vi "IR_Correction.vi"(1 "X Rate":bool=TRUE, 2 "X_Rotate Rate":bool=TRUE, 3 "Y Rate":bool=TRUE, 4 "Y_Rotate Rate":bool=TRUE, 5 "Mode":enum16{"LF", "LB", "RF", "RB"}(ring), 11 "error in":errorcluster, 12 "width":bool) -> (15 "error out":errorcluster)   [LabVIEW 2019]
uses:
  <vilib>/Platform/TimedLoop/XDataNode/timing_clust.ctl
  <vilib>/Platform/TimedLoop/XDataNode/nitl_modes.ctl
  <vilib>/Platform/TimedLoop/XDataNode/wakeup.ctl
  WSCbot_V3_Toolkit.lvlibp/WSCBOTV3_Toolkit/Sensor/LowLevel/IR_Chanel.ctl
  WSCbot_V3_Toolkit.lvlibp/WSCBOTV3_Toolkit/System/LowLevel/EMS.vi
  <vilib>/platform/TimedLoop/XDataNode/XDataNode.xnode
  <vilib>/Platform/TimedLoop/XDataNode/XDNodeRunTimeDep.lvlib
  WSCbot_V3_Toolkit.lvlibp
panel:
  out "X_Rotate IR":bool
  out "X_Rotate IR":dbl
  in  "Power Rate":dbl
  out "4xMotor":dbl[](graph)
  out "ENC":dbl[](graph)
  out "Waveform Chart 2":T1(graph)
  out "IR":T2
  out "Y_Rotate IR":dbl
  out "X Position IR":dbl
  out "Y Position IR":dbl
  out "Y_Rotate IR":bool
  out "X Position IR":bool
  out "Y Position IR":bool
  in  "Stop":bool
  out "result":bool
  out "Numeric":i32
  out "coerced(x)":dbl
  out "Boolean":bool
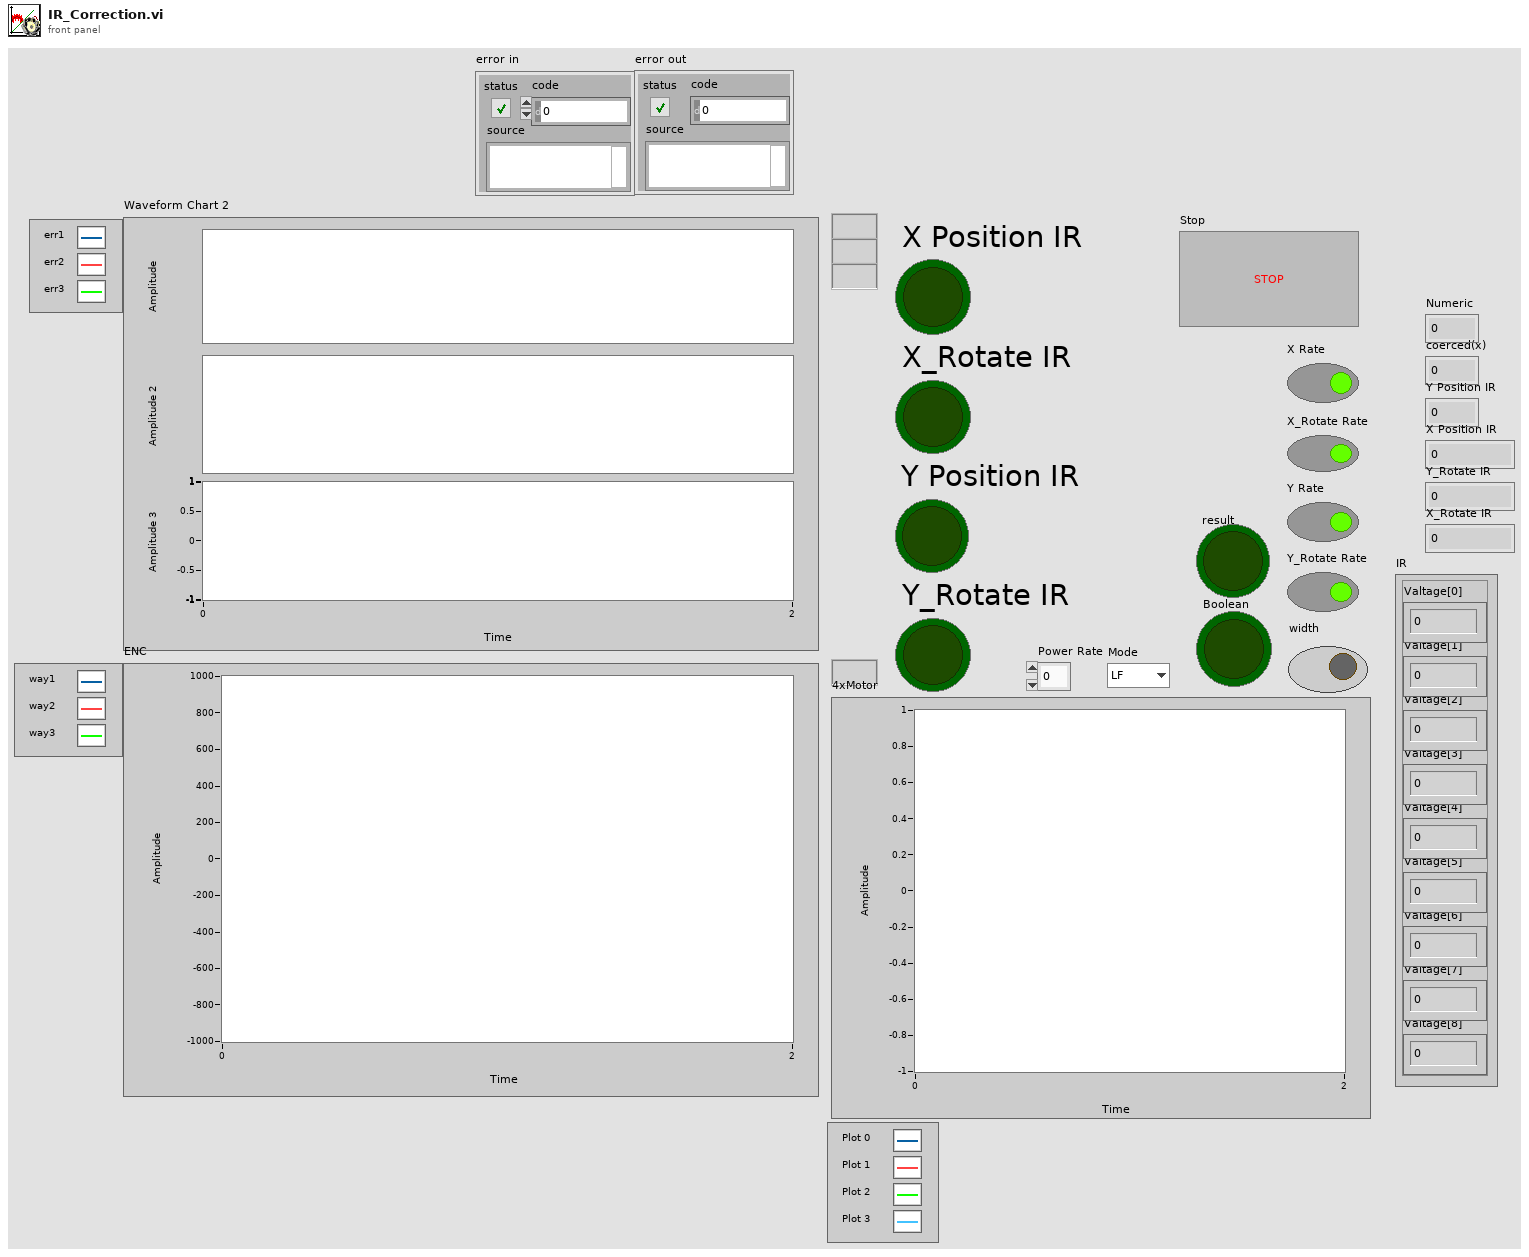
[diagram p1: front panel]
types:
  T1 = cluster{"Valtage[0]":dbl, "Valtage[1]":dbl, "Valtage[2]":dbl}
  T2 = cluster{"Valtage[0]":dbl, "Valtage[1]":dbl, "Valtage[2]":dbl, "Valtage[3]":dbl, "Valtage[4]":dbl, "Valtage[5]":dbl, "Valtage[6]":dbl, "Valtage[7]":dbl, "Valtage[8]":dbl}
  T3 = typedef "WSCbot_V3_Toolkit.lvlibp/IR_Chanel.ctl" = enum16{"IR_LF", "IR_LB", "IR_BL", "IR_BR", "IR_RB", "IR_RF", "IR_FR", "IR_FL"}
  T4 = typedef "XDNodeRunTimeDep.lvlib/timing_clust.ctl" = cluster{"Expected End [f-1]":u64, "Actual End [f-1]":u64, "Finished Late? [f-1]":bool, "Expected End [i-1]":u64, "Actual End [i-1]":u64, "Finished Late? [i-1]":bool, "Expected Start [i]":u64, "Actual Start [i]":u64, "Expected Start [f]":u64, "Actual Start [f]":u64, "Source Name":string, "Structure Name":string, "Period":i64, "Deadline":i64, "Offset":i64, "Start":i64, "Priority":i32, "Timeout":i32, "Mode":T5, "Wakeup Reason":T6, "Error":errorcluster, "Source Type":string, "Secondary Source Type":string, "Global End Time":u64, "Global Start Time":u64, "Frame Duration":u64, "Iteration Duration":u64, "Assigned CPU":i32, "I/O Scan Engine Mode":u32}
  T5 = typedef "XDNodeRunTimeDep.lvlib/nitl_modes.ctl" = enum32{"No Change", "Process missed periods, maintain original phase", "Discard missed periods, maintain original phase", "Process missed periods, ignore original phase", "Discard missed periods, ignore original phase"}
  T6 = typedef "XDNodeRunTimeDep.lvlib/wakeup.ctl" = enum32{"Normal", "Aborted", "Asynchronous wakeup", "Timing source error", "Timed loop error", "Timeout"}
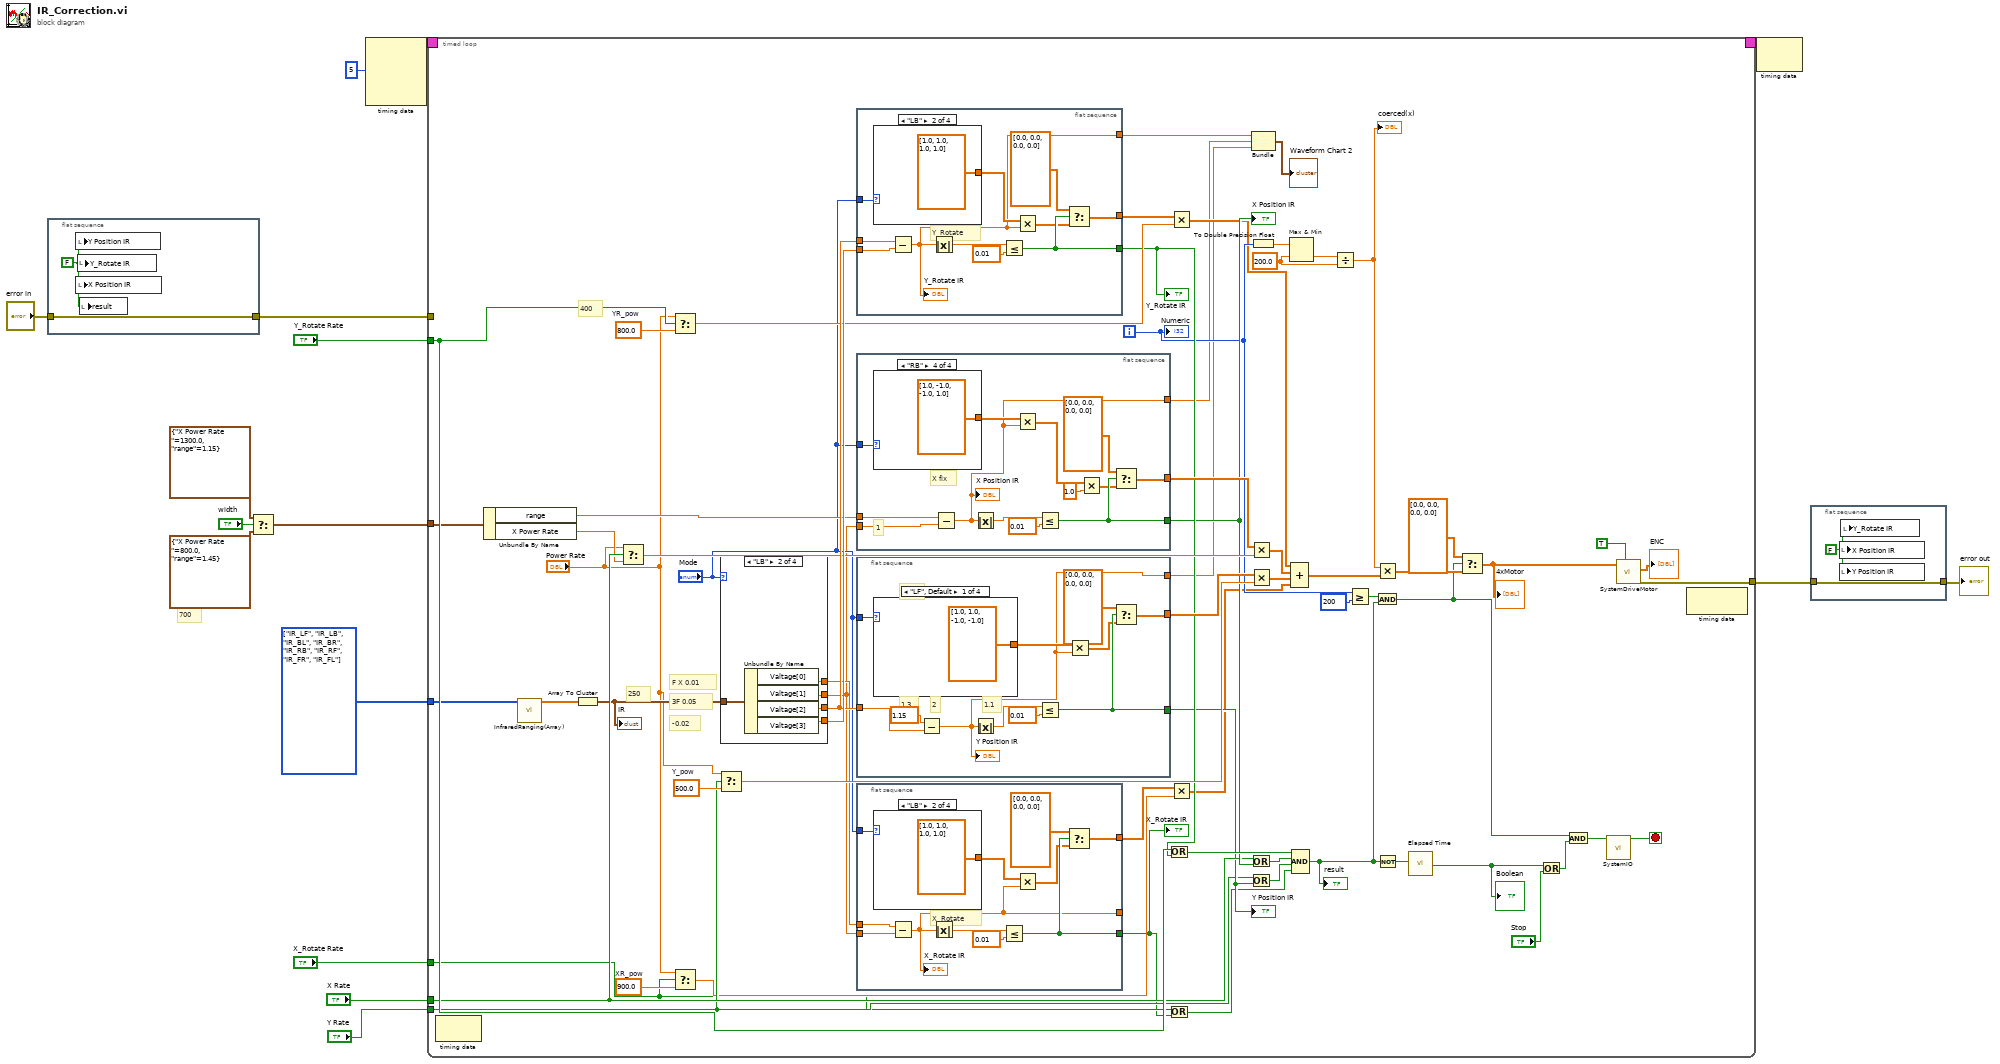
[diagram p0: block diagram]
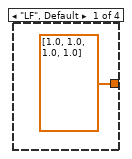
[diagram p2: hidden frame]
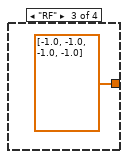
[diagram p3: hidden frame]
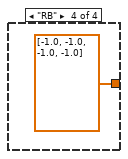
[diagram p4: hidden frame]
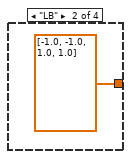
[diagram p5: hidden frame]
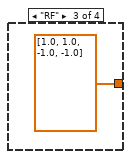
[diagram p6: hidden frame]
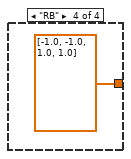
[diagram p7: hidden frame]
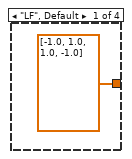
[diagram p8: hidden frame]
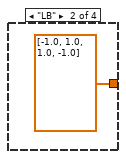
[diagram p9: hidden frame]
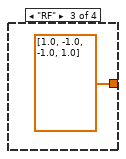
[diagram p10: hidden frame]
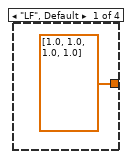
[diagram p11: hidden frame]
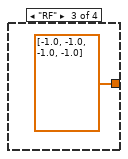
[diagram p12: hidden frame]
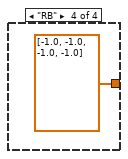
[diagram p13: hidden frame]
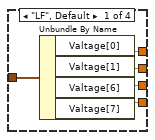
[diagram p14: hidden frame]
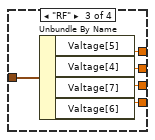
[diagram p15: hidden frame]
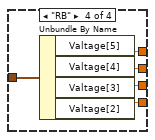
[diagram p16: hidden frame]
diagram:
  w4 = T3[] [enum."IR_LF", enum."IR_LB", enum."IR_BL", enum."IR_BR", enum."IR_RB", enum."IR_RF", enum."IR_FR", enum."IR_FL"] items=["IR_LF", "IR_LB", "IR_BL", "IR_BR", "IR_RB", "IR_RF", "IR_FR", "IR_FL"] ("IR_Chanel")
  # "700"
  n1 = flat-sequence {
    tunnel: "error in" -> [w18]
    tunnel: [w18] -> w3
    frame #0 {
      w17 = FALSE
      n2 = local write "Y Position IR"(w17) -> ()
      n3 = local write "X Position IR"(w17) -> ()
      n4 = local write "Y_Rotate IR"(w17) -> ()
      n5 = local write "result"(w17) -> ()
    }
  }
  n6 = Select(t=cluster{"X Power Rate ":dbl, "range":dbl} {"X Power Rate "=1300.0, "range"=1.15}, s="width", f=cluster{"X Power Rate ":dbl, "range":dbl} {"X Power Rate "=800.0, "range"=1.45}) -> (s? t:f=w8:cluster{"X Power Rate ":dbl, "range":dbl})
  n7 = node-c288(i64 5 ("Period")) -> (w16:T4)  [unwired: 3 in]
  n8 = timed-loop {
    timing: w16 -> [_]
    timing-out: [_] -> w15
    tunnel: w3 -> [_]
    tunnel: [w51] -> w1
    tunnel: "Y_Rotate Rate" -> [w65]
    tunnel: "X Rate" -> [w61]
    tunnel: "Y Rate" -> [w58]
    tunnel: w8 -> [w56]
    tunnel: w4 -> [w45]
    tunnel: "X_Rotate Rate" -> [w21]
    i -> [w40]
    stop <- w50 stop-if-true
    w28 = 900.0  # XR_pow
    w42 = 200.0 ("y")
    w67 = 500.0  # Y_pow
    w70 = 800.0  # YR_pow
    # "250"
    # "400"
    # "3F 0.05"
    # "F X 0.01"
    # "-0.02"
    n9 = node-c288() -> ()  [unwired: 1 in, 1 out]
    n10 = Unbundle By Name(w56) -> ("range"=w55:dbl, "X Power Rate"=w54:dbl)
    n11 = call "InfraredRanging(Array).vi"("IR_Chanel"=w45) -> ("Valtage"=w47:dbl[])  [unwired: 9 in, 1 out]
    n12 = Array To Cluster(array=w47) -> (cluster=w46:T2)
    "IR" <- w46
    n13 = Select(t="Power Rate", s=w61, f=w54) -> (s? t:f=w68:dbl)
    n14 = Select(t="Power Rate", s=w65, f=w70) -> (s? t:f=w69:dbl)
    n15 = Select(t="Power Rate", s=w21, f=w28) -> (s? t:f=w27:dbl)
    n16 = Select(t="Power Rate", s=w58, f=w67) -> (s? t:f=w66:dbl)
    n17 = case shown="\"LB\"" "Mode" {
      tunnel: [w150 w155 w159 w164] -> w82
      tunnel: [w149 w154 w160 w165] -> w83
      tunnel: [w152 w156 w161 w166] -> w23
      tunnel: w46 -> [w151 w157 w162 w167]
      tunnel: [w148 w153 w158 w163] -> w24
      frame "LF", Default {
        n18 = Unbundle By Name(w151) -> ("Valtage[0]"=w148:dbl, "Valtage[1]"=w152:dbl, "Valtage[6]"=w150:dbl, "Valtage[7]"=w149:dbl)
      }
      frame "LB" {
        n19 = Unbundle By Name(w157) -> ("Valtage[0]"=w153:dbl, "Valtage[1]"=w156:dbl, "Valtage[2]"=w155:dbl, "Valtage[3]"=w154:dbl)
      }
      frame "RF" {
        n20 = Unbundle By Name(w162) -> ("Valtage[5]"=w158:dbl, "Valtage[4]"=w161:dbl, "Valtage[7]"=w159:dbl, "Valtage[6]"=w160:dbl)
      }
      frame "RB" {
        n21 = Unbundle By Name(w167) -> ("Valtage[5]"=w163:dbl, "Valtage[4]"=w166:dbl, "Valtage[3]"=w164:dbl, "Valtage[2]"=w165:dbl)
      }
    }
    n22 = flat-sequence {
      tunnel: w82 -> [w141]
      tunnel: w83 -> [w140]
      tunnel: "Mode" -> [w139]
      tunnel: [w137] -> w64
      tunnel: [w134] -> w81
      tunnel: [w131] -> w36
      frame #0 {
        # "Y_Rotate"
        n23 = case shown="\"LB\"" w139 {
          tunnel: [dbl[] [1.0, 1.0, 1.0, 1.0] dbl[] [1.0, 1.0, 1.0, 1.0] dbl[] [-1.0, -1.0, -1.0, -1.0] dbl[] [-1.0, -1.0, -1.0, -1.0]] -> w133
          frame "LF", Default {
          }
          frame "LB" {
          }
          frame "RF" {
          }
          frame "RB" {
          }
        }
        n24 = Subtract(x=w141, y=w140) -> (x-y=w131:dbl)
        "Y_Rotate IR" <- w131
        n25 = Absolute Value(x=w131) -> (abs(x)=w132:dbl)
        n26 = Less Or Equal?(x=w132, y=0.01) -> (x <= y?=w137:bool)
        n27 = Multiply(x=w133, y=w131) -> (x*y=w136:dbl[])
        n28 = Select(t=dbl[] [0.0, 0.0, 0.0, 0.0], s=w137, f=w136) -> (s? t:f=w134:dbl[])
      }
    }
    n29 = flat-sequence {
      tunnel: w23 -> [w126]
      tunnel: "Mode" -> [w125]
      tunnel: [w120] -> w62
      tunnel: [w117] -> w80
      tunnel: w55 -> [w116]
      tunnel: [w114] -> w35
      frame #0 {
        # "1"
        # "X fix"
        n30 = case shown="\"RB\"" w125 {
          tunnel: [dbl[] [-1.0, 1.0, 1.0, -1.0] dbl[] [-1.0, 1.0, 1.0, -1.0] dbl[] [1.0, -1.0, -1.0, 1.0] dbl[] [1.0, -1.0, -1.0, 1.0]] -> w123
          frame "LF", Default {
          }
          frame "LB" {
          }
          frame "RF" {
          }
          frame "RB" {
          }
        }
        n31 = Subtract(x=w116, y=w126) -> (x-y=w114:dbl)
        "X Position IR" <- w114
        n32 = Absolute Value(x=w114) -> (abs(x)=w115:dbl)
        n33 = Multiply(x=w123, y=w114) -> (x*y=w122:dbl[])
        n34 = Less Or Equal?(x=w115, y=0.01) -> (x <= y?=w120:bool)
        n35 = Multiply(x=w122, y=1.0) -> (x*y=w119:dbl[])
        n36 = Select(t=dbl[] [0.0, 0.0, 0.0, 0.0], s=w120, f=w119) -> (s? t:f=w117:dbl[])
      }
    }
    n37 = flat-sequence {
      tunnel: "Mode" -> [w109]
      tunnel: w82 -> [w108]
      tunnel: [w105] -> w59
      tunnel: [w102] -> w79
      tunnel: [w99] -> w34
      frame #0 {
        # "1.1"
        # "1.3"
        # "2"
        # "Y fix"
        n38 = case shown="\"LF\", Default" w109 {
          tunnel: [dbl[] [1.0, 1.0, -1.0, -1.0] dbl[] [-1.0, -1.0, 1.0, 1.0] dbl[] [1.0, 1.0, -1.0, -1.0] dbl[] [-1.0, -1.0, 1.0, 1.0]] -> w106
          frame "LF", Default {
          }
          frame "LB" {
          }
          frame "RF" {
          }
          frame "RB" {
          }
        }
        n39 = Subtract(x=1.15 ("f"), y=w108) -> (x-y=w99:dbl)
        "Y Position IR" <- w99
        n40 = Absolute Value(x=w99) -> (abs(x)=w100:dbl)
        n41 = Less Or Equal?(x=w100, y=0.01) -> (x <= y?=w105:bool)
        n42 = Multiply(x=w106, y=w99) -> (x*y=w104:dbl[])
        n43 = Select(t=dbl[] [0.0, 0.0, 0.0, 0.0], s=w105, f=w104) -> (s? t:f=w102:dbl[])
      }
    }
    n44 = flat-sequence {
      tunnel: w24 -> [w94]
      tunnel: w23 -> [w93]
      tunnel: "Mode" -> [w92]
      tunnel: [w90] -> w20
      tunnel: [w87] -> w26
      tunnel: [w84] -> _
      frame #0 {
        # "X_Rotate"
        n45 = case shown="\"LB\"" w92 {
          tunnel: [dbl[] [1.0, 1.0, 1.0, 1.0] dbl[] [1.0, 1.0, 1.0, 1.0] dbl[] [-1.0, -1.0, -1.0, -1.0] dbl[] [-1.0, -1.0, -1.0, -1.0]] -> w86
          frame "LF", Default {
          }
          frame "LB" {
          }
          frame "RF" {
          }
          frame "RB" {
          }
        }
        n46 = Subtract(x=w94, y=w93) -> (x-y=w84:dbl)
        "X_Rotate IR" <- w84
        n47 = Absolute Value(x=w84) -> (abs(x)=w85:dbl)
        n48 = Less Or Equal?(x=w85, y=0.01) -> (x <= y?=w90:bool)
        n49 = Multiply(x=w86, y=w84) -> (x*y=w89:dbl[])
        n50 = Select(t=dbl[] [0.0, 0.0, 0.0, 0.0], s=w90, f=w89) -> (s? t:f=w87:dbl[])
      }
    }
    n51 = Or(x=w65, y=w64) -> (x .or. y?=w63:bool)
    n52 = Or(x=w21, y=w20) -> (x .or. y?=w19:bool)
    n53 = Multiply(x=w81, y=w69) -> (x*y=w39:dbl[])
    n54 = Multiply(x=w26, y=w27) -> (x*y=w25:dbl[])
    n55 = Multiply(x=w80, y=w68) -> (x*y=w38:dbl[])
    n56 = Multiply(x=w79, y=w66) -> (x*y=w37:dbl[])
    n57 = Or(x=w61, y=w62) -> (x .or. y?=w60:bool)
    n58 = Or(x=w58, y=w59) -> (x .or. y?=w22:bool)
    n59 = Bundle(w36, w35, w34) -> (→"Waveform Chart 2":cluster{dbl, dbl, dbl})  [unwired: 1 in]
    n60 = To Double Precision Float(number=w40) -> (double precision float=w44:dbl)
    n61 = Max & Min(x=w44, y=w42) -> (min(x,y)=w43:dbl)  [unwired: 1 out]
    n62 = Compound Arithmetic op=ADD(w39, w38, w37, w25) -> (w75:dbl[])
    n63 = Compound Arithmetic op=AND(w63, w60, w22, w19) -> (w71:bool)
    "result" <- w71
    n64 = Divide(x=w43, y=w42) -> (x/y=w41:dbl)
    "coerced(x)" <- w41
    n65 = Greater Or Equal?(x=w40, y=200) -> (x >= y?=w76:bool)
    n66 = Multiply(x=w41, y=w75) -> (x*y=w74:dbl[])
    n67 = And(x=w76, y=w71) -> (x .and. y?=w53:bool)
    n68 = Not(x=w71) -> (.not. x?=w72:bool)
    n69 = call "Elapsed Time"("Reset"=w72) -> ("Time has Elapsed"=w57:bool)  [unwired: 11 in, 7 out]
    "Boolean" <- w57
    n70 = Select(t=dbl[] [0.0, 0.0, 0.0, 0.0], s=w53, f=w74) -> (s? t:f=w31:dbl[])
    "4xMotor" <- w31
    n71 = Or(x=w57, y="Stop") -> (x .or. y?=w52:bool)
    n72 = And(x=w53, y=w52) -> (x .and. y?=w49:bool)
    n73 = call-poly "SystemIO.vi"("ProgramStop"=w49) -> ("EMS"=w50:bool)  [unwired: 9 in, 1 out]
    n74 = call "SystemDriveMotor.vi"("Enable?"=TRUE, "4xMotor(deg/s)"=w31) -> ("error out"=w51:errorcluster, "ENC (deg)"=→"ENC":dbl[])  [unwired: 8 in]
    n75 = node-c288() -> ()  [unwired: 1 in, 1 out]
    "Y_Rotate IR" <- w64
    "X Position IR" <- w62
    "Y Position IR" <- w59
    "Numeric" <- w40
    "X_Rotate IR" <- w20
  }
  n76 = node-c288(w15) -> ()  [unwired: 1 out]
  n77 = flat-sequence {
    tunnel: w1 -> [w168]
    tunnel: [w168] -> w5
    frame #0 {
      w169 = FALSE ("Rotate IR")
      n78 = local write "X Position IR"(w169) -> ()
      n79 = local write "Y Position IR"(w169) -> ()
      n80 = local write "Y_Rotate IR"(w169) -> ()
    }
  }
  "error out" <- w5
